vi "Iterative File Write.vi"(5 "Username":string, 6 "Password":string, 7 "Address":string, 8 "Error In":errorcluster) -> (0 "Error Out":errorcluster)   [LabVIEW 2018, in "Tests.lvlib" / "SFTP File.lvlib"]
uses:
  SFTP File.lvlib
  src/Toolkit/API/SFTP File/API/Typedefs/Flags.ctl
  src/Toolkit/API/Typedefs/Permissions.ctl
  src/Toolkit/API/Typedefs/Modes.ctl
  src/Toolkit/API/SFTP Attributes/SFTP Attributes.lvclass/SFTP Attributes.ctl
  src/Toolkit/API/SSH/SSH.lvclass/SSH.ctl
  src/Toolkit/API/SSH/Utility/Read Shared Library.vi
  src/Toolkit/API/SFTP Attributes/Support/Create from SFTP File.vi
  src/Toolkit/Support/Check Status.vi
  src/Toolkit/API/SFTP Attributes/Support/Destroy to SFTP File.vi
  src/Toolkit/API/SFTP File/SFTP File.lvclass
  src/Toolkit/Toolkit.lvlib
  <vilib>/addons/_JKI Toolkits/Caraya/classes/Test/Test.lvclass
  <vilib>/addons/_JKI Toolkits/Caraya/classes/Assert/Assert.lvclass
  src/Toolkit/API/SFTP Attributes/SFTP Attributes.lvclass
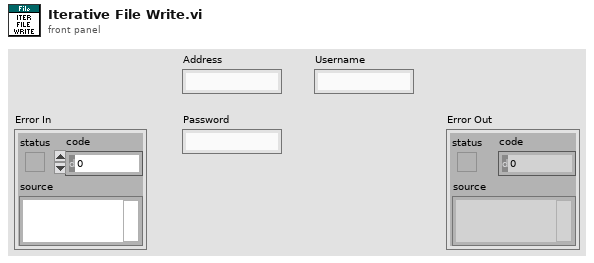
[diagram p1: front panel]
types:
  T1 = enum16{"open", "replace", "create", "open or create", "replace or create", "replace or create with confirmation"}
  T2 = typedef "Toolkit.lvlib/Permissions.ctl" = cluster{"Owner":T3, "Group":T3, "Others":T3}
  T3 = typedef "Toolkit.lvlib/Modes.ctl" = cluster{"Read":bool, "Write":bool, "Execute":bool}
  T4 = typedef "Toolkit.lvlib/SFTP File.lvclass/Flags.ctl" = cluster{"Read":bool, "Write":bool, "Append":bool, "Create":bool, "Truncate":bool, "Exclude":bool}
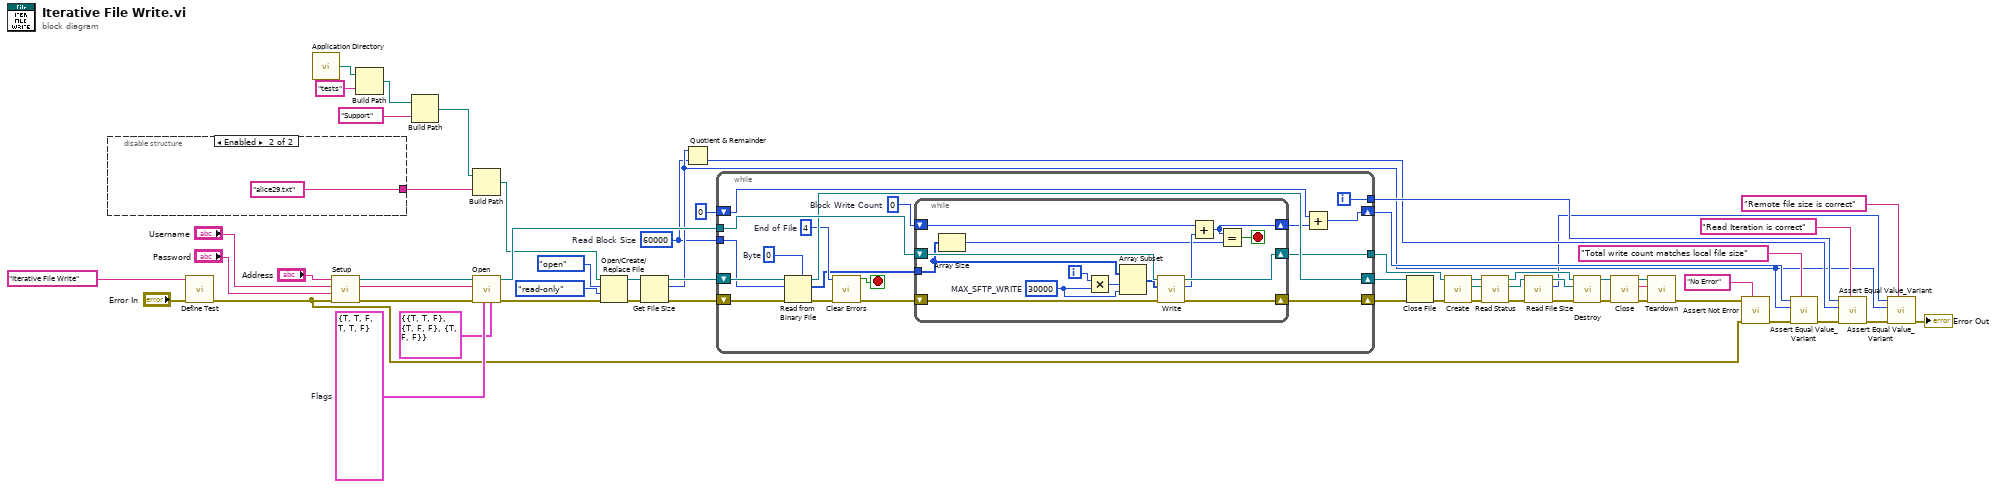
[diagram p0: block diagram]
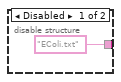
[diagram p2: hidden frame]
diagram:
  w3 = i64 60000  # Read Block Size
  w54 = T4 {"Read"=TRUE, "Write"=TRUE, "Append"=FALSE, "Create"=TRUE, "Truncate"=TRUE, "Exclude"=FALSE}  # Flags
  n1 = disable-structure "Diagram Disable Structure" shown="Enabled" {
    disable-tunnel: ["EColi.txt" ("name or relative path") "alice29.txt" ("name or relative path")] -> w36
    frame Disabled {
    }
    frame Enabled {
    }
  }
  n2 = call <vilib>:"Define Test.vi"("error in (no error)"="Error In", "Label (VI Title)"="Iterative File Write") -> ("error out"=w32:errorcluster)  [unwired: 9 in]
  n3 = call <vilib>:"Application Directory.vi"() -> ("Application Directory"=w44:path)
  n4 = call "Setup.vi"("Error In"=w32, "Password"="Password", "Username"="Username", "Address"="Address") -> ("Error Out"=w53:errorcluster, "Temporary File"=w45:string, "SFTP"=w56:refnum<class "SFTP.lvclass">)  [unwired: 5 in]
  n5 = Build Path(base path=w44, name or relative path="tests") -> (appended path=w42:path)
  n6 = Build Path(base path=w42, name or relative path="Support") -> (appended path=w40:path)
  n7 = Build Path(base path=w40, name or relative path=w36) -> (appended path=w39:path)
  n8 = call "Open.vi"("Permissions"=T2 {"Owner"={"Read"=TRUE, "Write"=TRUE, "Execute"=FALSE}, "Group"={"Read"=TRUE, "Write"=FALSE, "Execute"=FALSE}, "Others"={"Read"=TRUE, "Write"=FALSE, "Execute"=FALSE}}, "Flags"=w54, "Error In"=w53, "Remote Path"=w45, "SFTP"=w56) -> ("Error Out"=w29:errorcluster, "SFTP File"=w55:refnum<class "SFTP File.lvclass">)  [unwired: 5 in]
  n9 = Open/Create/Replace File(file path (use dialog)=w39, error in=w29, operation (0:open)=T1."open", access (0:read/write)=enum16{"read/write", "read-only", "write-only"}."read-only") -> (refnum out=w46:refnum<file>, error out=w26:errorcluster)  [unwired: 2 in, 1 out]
  n10 = Get File Size(file=w46, error in=w26) -> (refnum out=w27:refnum<file>, size (in bytes)=w4:i64, 0:w25:errorcluster)
  n11 = Quotient & Remainder(x=w4, y=w3) -> (floor(x/y)=w19:i64)  [unwired: 1 out]
  n12 = while {
    tunnel: w55 -> [w79]
    tunnel: w3 -> [w65]
    shift-right: [w76] -> w38
    shift-left: w27 -> [w78]
    shift-right: [w68] -> w37
    shift-left: w25 -> [w77]
    tunnel: [w69] -> w1
    shift-right: [w66] -> w24
    shift-left: i64 0 -> [w72]
    tunnel: [w70] -> w20
    i -> [w70]
    stop <- w64 stop-if-true
    w63 = i64 0  # Block Write Count
    w71 = u8 0  # Byte
    w74 = 4  # End of File
    n13 = Read from Binary File(5:w71, 8:w77, 10:w65, 11:w78) -> (0:w75:errorcluster, 2:w67:u8[], 3:w76:refnum<file>)  [unwired: 2 in, 1 out]
    n14 = call <vilib>:"Clear Errors.vi"("error in (no error)"=w75, "specific error code to clear (0: all)"=w74) -> ("error out"=w73:errorcluster, "specific error cleared?"=w64:bool)  [unwired: 4 in]
    n15 = while {
      tunnel: w67 -> [w84]
      shift-right: [w91] -> w69
      shift-left: w79 -> [w93]
      shift-right: [w90] -> w68
      shift-left: w73 -> [w92]
      shift-right: [w87] -> w62
      shift-left: w63 -> [w89]
      i -> [w83]
      stop <- w85 stop-if-true
      w81 = 30000  # MAX_SFTP_WRITE
      n16 = Array Size(array=w84) -> (size(s)=w86:i32)
      n17 = Multiply(x=w83, y=w81) -> (x*y=w82:i32)
      n18 = Array Subset(array=w84, index=w82, length=w81) -> (w80:u8[])
      n19 = call "Write.vi"("Error In"=w92, "Data"=w80, "SFTP File In"=w93) -> ("Error Out"=w90:errorcluster, "Count"=w88:i64, "SFTP File Out"=w91:refnum<class "SFTP File.lvclass">)  [unwired: 6 in]
      n20 = Add(x=w89, y=w88) -> (x+y=w87:i64)
      n21 = Equal?(x=w87, y=w86) -> (x = y?=w85:bool)
    }
    n22 = Add(x=w72, y=w62) -> (x+y=w66:i64)
  }
  n23 = Close File(refnum=w38, error in=w37) -> (error out=w2:errorcluster)  [unwired: 1 out]
  n24 = call-poly "Create.vi"("Error In"=w2, "SFTP File In"=w1) -> ("Error Out"=w16:errorcluster, "SFTP Attributes"=w17:refnum<class "SFTP Attributes.lvclass">, "SFTP File Out"=w18:refnum<class "SFTP File.lvclass">)  [unwired: 7 in]
  n25 = call "Read Status.vi"("Error In"=w16, "Attributes In"=w17, "SFTP File In"=w18) -> ("Error Out"=w15:errorcluster, "Attributes Out"=w14:refnum<class "SFTP Attributes.lvclass">, "SFTP File Out"=w13:refnum<class "SFTP File.lvclass">)  [unwired: 6 in]
  n26 = call "Read File Size.vi"("Error In"=w15, "SFTP Attributes In"=w14) -> ("Error Out"=w11:errorcluster, "File Size"=w5:u64, "SFTP Attribute Out"=w12:refnum<class "SFTP Attributes.lvclass">)  [unwired: 7 in]
  n27 = call-poly "Destroy.vi"("Error In"=w11, "SFTP Attributes"=w12, "SFTP File In"=w13) -> ("Error Out"=w10:errorcluster, "SFTP File Out"=w9:refnum<class "SFTP File.lvclass">)  [unwired: 7 in]
  n28 = call "Close.vi"("Error In"=w10, "SFTP File"=w9) -> ("Error Out"=w50:errorcluster, "Remote Path"=w52:string, "SFTP"=w51:refnum<class "SFTP.lvclass">)  [unwired: 7 in]
  n29 = call "Teardown.vi"("Error In"=w50, "Temporary File"=w52, "SFTP"=w51) -> ("Error Out"=w33:errorcluster)  [unwired: 8 in]
  n30 = call <vilib>:"Assert Not Error.vi"("Label"="No Error", "error in (no error)"=w32, "Not Error?"=w33) -> ("error out"=w30:errorcluster)  [unwired: 8 in]
  n31 = call <vilib>:"Assert Equal Value_Variant.vi"("Label"="Total write count matches local file size", "error in (no error)"=w30, "Y"=w4, "X"=w24) -> ("error out"=w22:errorcluster)  [unwired: 7 in]
  n32 = call <vilib>:"Assert Equal Value_Variant.vi"("Label"="Read Iteration is correct", "error in (no error)"=w22, "Y"=w19, "X"=w20) -> ("error out"=w8:errorcluster)  [unwired: 7 in]
  n33 = call <vilib>:"Assert Equal Value_Variant.vi"("Label"="Remote file size is correct", "error in (no error)"=w8, "Y"=w4, "X"=w5) -> ("error out"=→"Error Out":errorcluster)  [unwired: 7 in]
